vi "Calibrate Timeouts 2 Ticks (uSMC).vi"(0 "Buttons Timeout 1 (ms)":u16, 1 "Reduce Current Timeout (ms)":u16, 5 "Buttons Timeout 2 (ms)":u16, 7 "Buttons Timeout 3 (ms)":u16, 9 "Buttons Timeout 4 (ms)":u16, 11 "Buttons Timeout Reset (ms)":u16, 12 "Buttons Timeout DblClick (ms)":u16) -> (3 "Reduce Current Timeout (ticks)":u16=6458, 4 "Buttons Timeout 1 (ticks)":u16=4262, 6 "Buttons Timeout 2 (ticks)":u16=12916, 8 "Buttons Timeout 3 (ticks)":u16=12916, 10 "Buttons Timeout 4 (ticks)":u16=12916, 14 "Buttons Timeout DblClick (ticks)":u16=1937, 15 "Buttons Timeout Reset (ticks)":u16=9687)   [LabVIEW 2010, in "SignalWriterMH110203USBStepperMotor.lvclass"]
uses:
  SignalWriterMH110203USBStepperMotor.lvclass
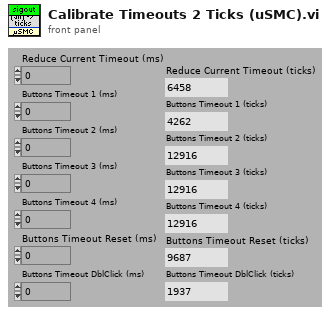
[diagram p1: front panel]
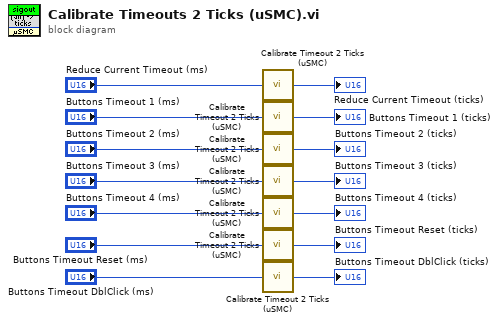
[diagram p0: block diagram]
diagram:
  n1 = call "Calibrate Timeout 2 Ticks (uSMC).vi"("Timeout (ms)"="Reduce Current Timeout (ms)") -> ("Timeout (Ticks)"=→"Reduce Current Timeout (ticks)":u16)
  n2 = call "Calibrate Timeout 2 Ticks (uSMC).vi"("Timeout (ms)"="Buttons Timeout 1 (ms)") -> ("Timeout (Ticks)"=→"Buttons Timeout 1 (ticks)":u16)
  n3 = call "Calibrate Timeout 2 Ticks (uSMC).vi"("Timeout (ms)"="Buttons Timeout 2 (ms)") -> ("Timeout (Ticks)"=→"Buttons Timeout 2 (ticks)":u16)
  n4 = call "Calibrate Timeout 2 Ticks (uSMC).vi"("Timeout (ms)"="Buttons Timeout 3 (ms)") -> ("Timeout (Ticks)"=→"Buttons Timeout 3 (ticks)":u16)
  n5 = call "Calibrate Timeout 2 Ticks (uSMC).vi"("Timeout (ms)"="Buttons Timeout 4 (ms)") -> ("Timeout (Ticks)"=→"Buttons Timeout 4 (ticks)":u16)
  n6 = call "Calibrate Timeout 2 Ticks (uSMC).vi"("Timeout (ms)"="Buttons Timeout Reset (ms)") -> ("Timeout (Ticks)"=→"Buttons Timeout Reset (ticks)":u16)
  n7 = call "Calibrate Timeout 2 Ticks (uSMC).vi"("Timeout (ms)"="Buttons Timeout DblClick (ms)") -> ("Timeout (Ticks)"=→"Buttons Timeout DblClick (ticks)":u16)
